vi "kt_numberArray.131125.vi"(8 "error in (no error)":errorcluster, 11 "Array In":dbl[][](array[numeric])) -> (0 "error out":errorcluster, 3 "Array Out":dbl[][](array[numeric]))   [LabVIEW 2013]
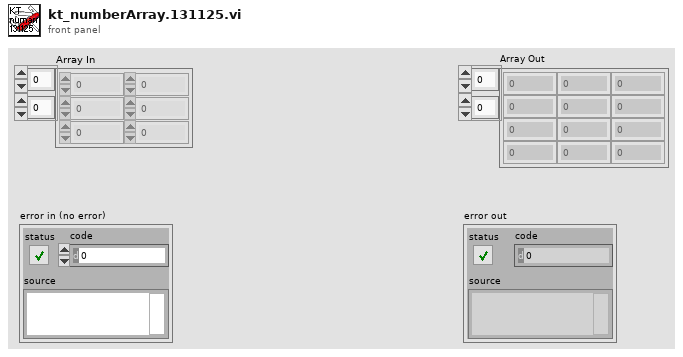
[diagram p1: front panel]
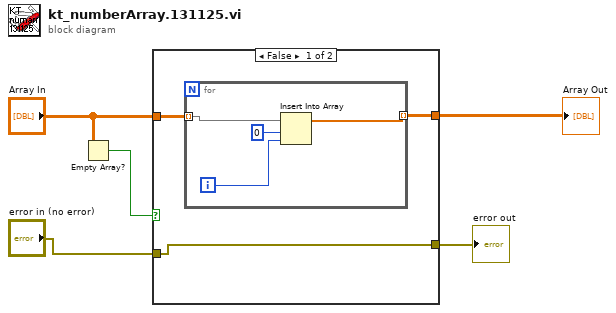
[diagram p0: block diagram]
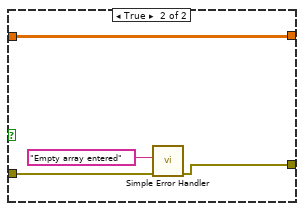
[diagram p2: hidden frame]
diagram:
  n1 = Empty Array?(array="Array In") -> (empty?=w3:bool)
  n2 = case shown="False" w3 {
    tunnel: "error in (no error)" -> [w8 w16]
    tunnel: [w8 w15] -> w4
    tunnel: "Array In" -> [w7 w13]
    tunnel: [w6 w13] -> w1
    frame False {
      n3 = for {
        tunnel: w7 -> [w12] mode=indexing
        tunnel: [w10] -> w6 mode=indexing
        i -> [w9]
        n4 = Insert Into Array(array=w12, index=0, new element=w9) -> (w10:dbl[])
      }
    }
    frame True {
      n5 = call <vilib>:"Simple Error Handler.vi"("error source (\" \")"="Empty array entered" ("error source (\" \")"), "error in (no error)"=w16) -> ("error out"=w15:errorcluster)  [unwired: 3 in, 4 out]
    }
  }
  "Array Out" <- w1
  "error out" <- w4
